vi "Rotate_DBL.vi"(7 "Direction of Rotation":T1, 8 "error in (no error)":errorcluster, 10 "Angle (degrees)":dbl, 11 "PolarVector in":refnum<class "PolarVector.lvclass">) -> (0 "error out":errorcluster, 3 "PolarVector out":refnum<class "PolarVector.lvclass">)   [LabVIEW 2013, in "PolarVector.lvclass"]
doc: "Takes in a PolarVector object, a direction of rotation and DBL value for angle of rotation. Outputs a new PolarVector object that has been rotated by the correct amount."
uses:
  PolarVector.lvclass
  TypeDefs/DirectionOfRotation.ctl
  PolarVector.lvclass/PolarVector.ctl
  Angles/Angle/Angle.lvclass
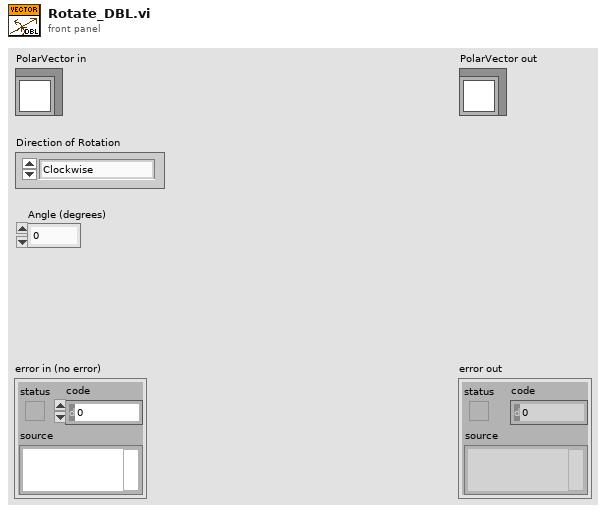
[diagram p1: front panel]
types:
  T1 = typedef "DirectionOfRotation.ctl" = enum16{"Clockwise", "Counter-Clockwise"}
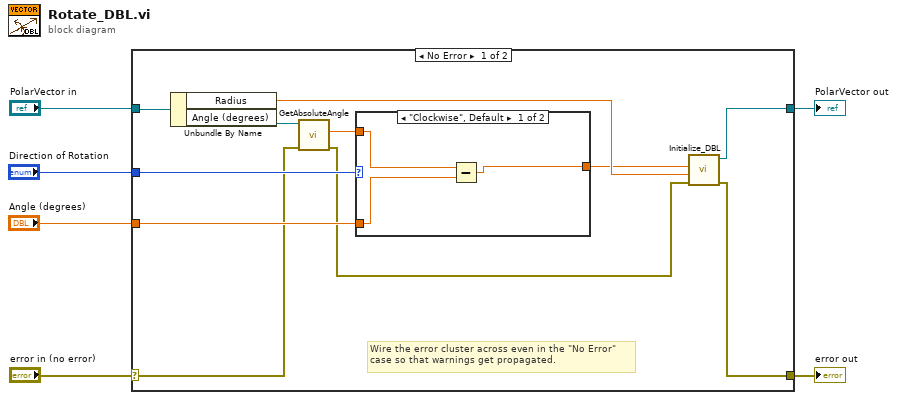
[diagram p0: block diagram]
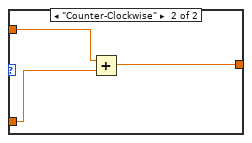
[diagram p2: hidden frame]
diagram:
  n1 = case shown="No Error" "error in (no error)" {
    selector: "error in (no error)" -> [w12 w25]
    tunnel: [w8 w25] -> w5
    tunnel: [w7 w24] -> w3
    tunnel: "PolarVector in" -> [w16 w24]
    tunnel: "Direction of Rotation" -> [w14 _]
    tunnel: "Angle (degrees)" -> [w17 _]
    frame No Error {
      # "Wire the error cluster across even in the \"No Error\"\ncase so that warnings get propagated."
      n2 = Unbundle By Name(w16) -> ("Radius"=w11:dbl, "Angle (degrees)"=w15:refnum<class "Angle.lvclass">)
      n3 = call "GetAbsoluteAngle.vi"("error in (no error)"=w12, "Angle in"=w15) -> ("error out"=w9:errorcluster, "Absolute angle (Deg.)"=w13:dbl)  [unwired: 8 in]
      n4 = case shown="\"Clockwise\", Default" w14 {
        tunnel: w17 -> [w19 w23]
        tunnel: w13 -> [w20 w22]
        tunnel: [w18 w21] -> w10
        frame "Clockwise", Default {
          n5 = Subtract(x=w20, y=w19) -> (x-y=w18:dbl)
        }
        frame "Counter-Clockwise" {
          n6 = Add(x=w22, y=w23) -> (x+y=w21:dbl)
        }
      }
      n7 = call "Initialize_DBL.vi"("error in (no error)"=w9, "Radius"=w11, "Angle (degrees)"=w10) -> ("error out"=w8:errorcluster, "PolarVector out"=w7:refnum<class "PolarVector.lvclass">)  [unwired: 7 in]
    }
    frame Error {
    }
  }
  "error out" <- w5
  "PolarVector out" <- w3
